vi "CRYNew View Global.vi"() -> ()   [LabVIEW 2013]
uses:
  Control/Graph Main Info Cluster.ctl
  <vilib>/Utility/miscctls.llb/LVRectTypeDef.ctl
panel:
  in  "g_GraphClicked":bool
  in  "g_WaitFlag":bool
  out "splitter_thickness":u32=4
  out "panel_offset":i32=3
  in  "Resize nID Array":i32[](array[numeric])
  out "bMouseMoveStarted":bool
  out "Data View Idx":i32
  out "Command Queue":i32[](array[numeric])
  in  "sMouseMoveVIEWTitle":string
  in  "Graph VritualBounds":T1
  in  "Graph VritualVIVisible":bool
  out "DV MarkSub Visible":bool
  in  "Parent Ref":refnum<vi>
  out "Data View Array Idx":i32
  in  "Graph Queue Name":string
  out "Data View Count":i32
  in  "AddGraphMenuVI":refnum<vi>
  in  "DV Virtual_sPos":string
  in  "DV MarkVIs":refnum<vi>[](array[refnum])
  in  "DV VirtualVI":refnum<vi>
  out "DV VirtualVisible":bool
  out "DV MarkVisible":bool
  in  "DV VirtualDoc VI":refnum<vi>
  out "DV ActiveDockVI Num":i32=-2
  in  "DView_idx_Array":i32[](array[numeric])
  in  "DataView_Global":T2[](array[typedef])
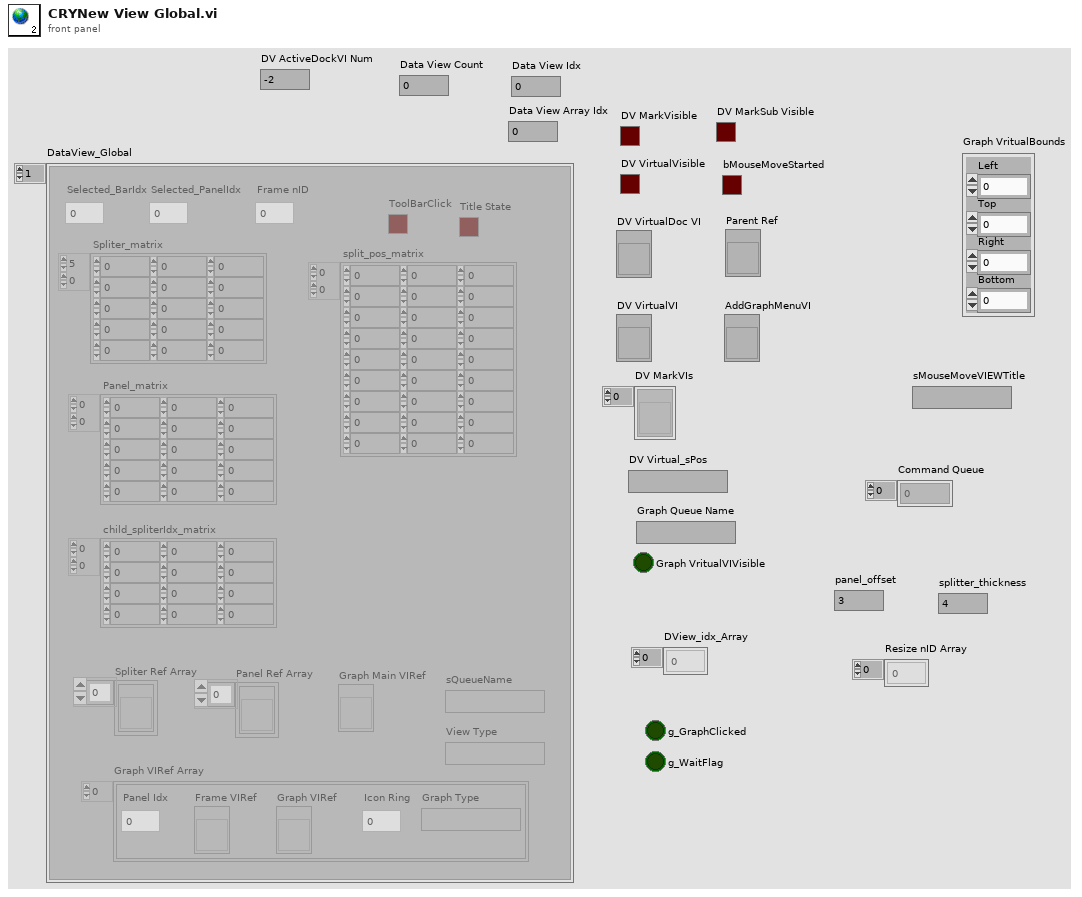
[diagram p1: front panel]
types:
  T1 = typedef "LVRectTypeDef.ctl" = cluster{"Left":i16, "Top":i16, "Right":i16, "Bottom":i16}
  T2 = typedef "Graph Main Info Cluster.ctl" = cluster{"Selected_BarIdx":i32, "Selected_PanelIdx":i32, "Graph Main VIRef":refnum<vi>, "ToolBarClick":bool, "Spliter Ref Array":refnum<vi>[], "Panel Ref Array":refnum<vi>[], "Spliter_matrix":i32[][], "Panel_matrix":i32[][], "child_spliterIdx_matrix":i32[][], "split_pos_matrix":i32[][], "Title State":bool, "sQueueName":string, "Frame nID":i32, "Graph VIRef Array":cluster{"Graph VIRef":refnum<vi>, "Panel Idx":i32, "Frame VIRef":refnum<vi>, "Icon Ring":i32, "Graph Type":string}[], "View Type":string}
diagram:
